vi "message c2s.vi"(0 "cluster":T1 {"id" format="%x"; "data" format="%x"}, 1 "add header? (F)":bool) -> (2 "string":string)   [LabVIEW 2024, in "atsj peakcan basic.lvlib"]
uses:
  atsj peakcan basic.lvlib
  message.ctl
  message type.ctl
  <vilib>/Utility/error.llb/whitespace.ctl
  <vilib>/Utility/error.llb/Trim Whitespace One-Sided.vi
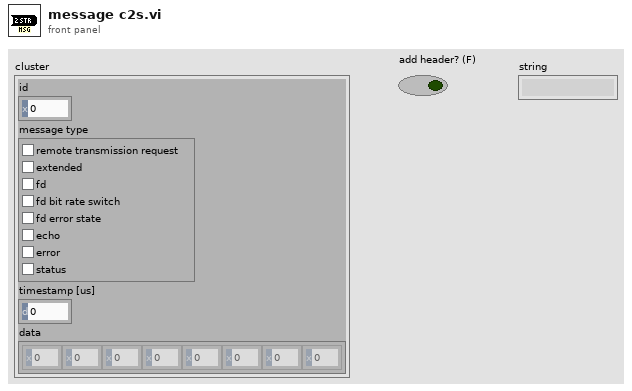
[diagram p1: front panel]
types:
  T1 = typedef "atsj peakcan basic.lvlib/message.ctl" = cluster{"id":u32, "message type":T2, "timestamp [us]":u64, "data":u8[]}
  T2 = typedef "atsj peakcan basic.lvlib/message type.ctl" = cluster{"remote transmission request ":bool, "extended":bool, "fd":bool, "fd bit rate switch":bool, "fd error state":bool, "echo":bool, "error":bool, "status":bool}
  T3 = typedef "whitespace.ctl" = u16
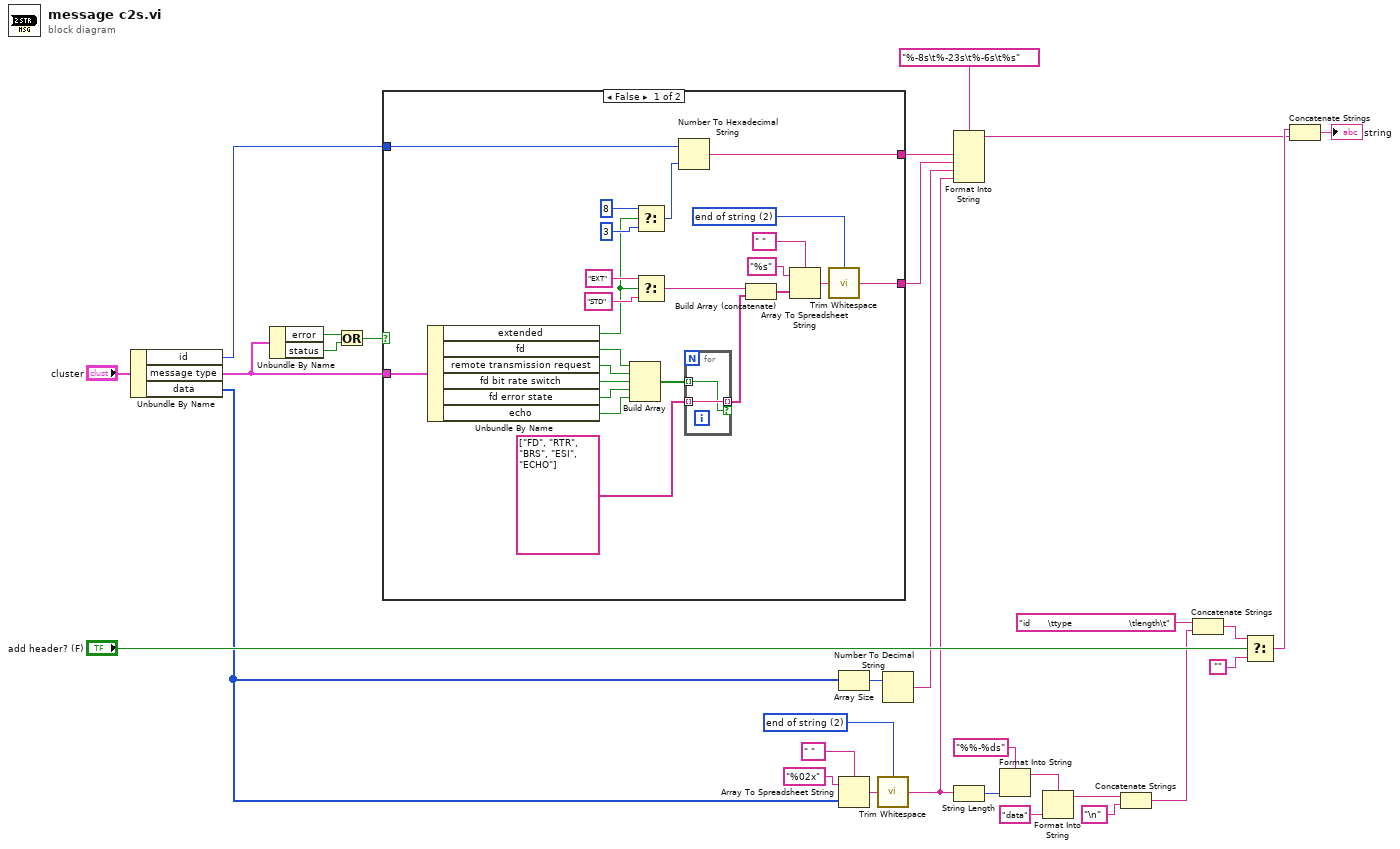
[diagram p0: block diagram]
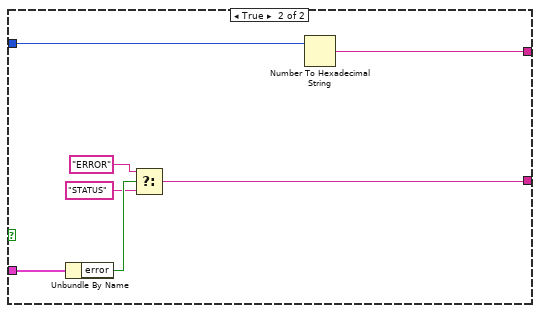
[diagram p2: hidden frame]
diagram:
  w24 = T3 2 items=["both", "start of string", "end of string"]
  n1 = Unbundle By Name("cluster") -> ("id"=w28:u32, "message type"=w4:T2, "data"=w21:u8[])
  n2 = Unbundle By Name(w4) -> ("error"=w3:bool, "status"=w2:bool)
  n3 = Or(x=w3, y=w2) -> (x .or. y?=w1:bool)
  n4 = case shown="False" w1 {
    tunnel: w4 -> [w54 w64]
    tunnel: w28 -> [w48 w59]
    tunnel: [w33 w58] -> w27
    tunnel: [w32 w60] -> w25
    frame False {
      w34 = T3 2 items=["both", "start of string", "end of string"]
      n5 = Unbundle By Name(w54) -> ("extended"=w41:bool, "fd"=w53:bool, "remote transmission request"=w52:bool, "fd bit rate switch"=w51:bool, "fd error state"=w50:bool, "echo"=w45:bool)
      n6 = Build Array(w53, w52, w51, w50, w45) -> (w49:bool[])
      n7 = Select(t=i16 8, s=w41, f=i16 3) -> (s? t:f=w46:i16)
      n8 = Select(t="EXT", s=w41, f="STD") -> (s? t:f=w40:string)
      n9 = Number To Hexadecimal String(1:w46, 2:w48) -> (0:w33:string)
      n10 = for {
        tunnel: w49 -> [w56] mode=indexing
        tunnel: string[] ["FD", "RTR", "BRS", "ESI", "ECHO"] -> [w57] mode=indexing
        tunnel: [w57] -> w39 mode=indexing if=w56
      }
      n11 = Build Array (concatenate)(w40, w39) -> (w36:string[])
      n12 = Array To Spreadsheet String(delimiter (Tab)=" ", array=w36, 3:"%s") -> (spreadsheet string=w35:string)
      n13 = call <vilib>:"Trim Whitespace.vi"("string"=w35, "location (both)"=w34) -> ("trimmed string"=w32:string)
    }
    frame True {
      n14 = Unbundle By Name(w64) -> ("error"=w63:bool)
      n15 = Select(t="ERROR", s=w63, f="STATUS") -> (s? t:f=w60:string)
      n16 = Number To Hexadecimal String(2:w59) -> (0:w58:string)  [unwired: 1 in]
    }
  }
  n17 = Array Size(array=w21) -> (size(s)=w16:i32)
  n18 = Array To Spreadsheet String(delimiter (Tab)=" ", array=w21, 3:"%02x") -> (spreadsheet string=w23:string)
  n19 = call <vilib>:"Trim Whitespace.vi"("string"=w23, "location (both)"=w24) -> ("trimmed string"=w14:string)
  n20 = Number To Decimal String(number=w16) -> (decimal integer string=w15:string)  [unwired: 1 in]
  n21 = Format Into String(format string="%-8s\t%-23s\t%-6s\t%s", w27, w25, w15, w14) -> (resulting string=w19:string)  [unwired: 2 in, 1 out]
  n22 = String Length(string=w14) -> (length=w12:i32)
  n23 = Format Into String(format string="%%-%ds", w12) -> (resulting string=w11:string)  [unwired: 2 in, 1 out]
  n24 = Format Into String(format string=w11, "data") -> (resulting string=w9:string)  [unwired: 2 in, 1 out]
  n25 = Concatenate Strings(w9, "\n") -> (w6:string)
  n26 = Concatenate Strings("id      \ttype                   \tlength\t", w6) -> (w5:string)
  n27 = Select(t=w5, s="add header? (F)", f="") -> (s? t:f=w20:string)
  n28 = Concatenate Strings(w20, w19) -> (→"string":string)
